vi "Signal generator (subVI).vi"(6 "DSA settings":T1={"function"=enum."Frequency response", "baseband span"=20000.0, "window"=enum."Hanning", "resolution (# of lines)"=800}, 7 "reset signal":bool, 8 "error in (no error)":errorcluster, 11 "signal generator":T2={"signal type"=enum."Uniform White noise", "frequency"=200.0, "amplitude"=1.0}) -> (0 "error out":errorcluster, 3 "signal out":waveform(dbl))   [LabVIEW 2020]
doc: "Generate typical test signal from the following choices: Sine wave, Square wave, Triangle wave, Sawtooth wave, Uniform White Noise, Gaussian White Noise, Periodic Random Noise (PRN), and Chirp."
uses:
  <vilib>/measure/NI_MABase.lvlib
  <vilib>/Analysis/NI_AALBase.lvlib
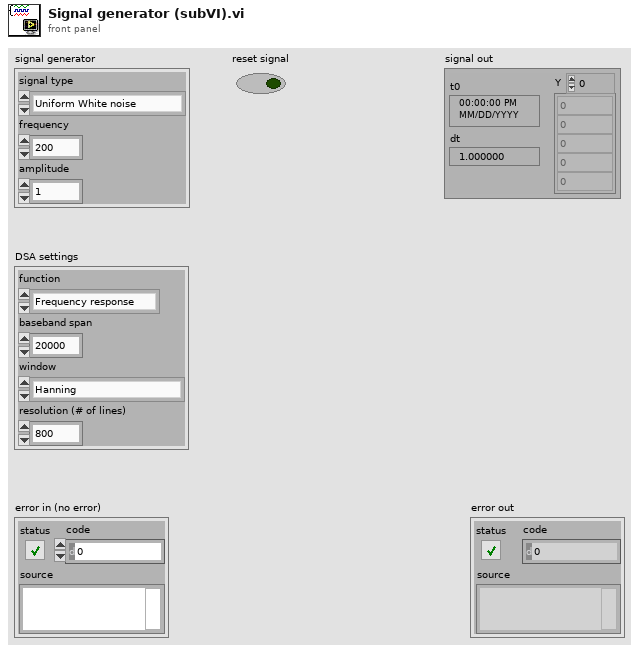
[diagram p1: front panel]
types:
  T1 = cluster{"function":enum16{"Windowed time", "Power Spectrum", "FFT (Mag-Phase)", "Cross Power spectrum", "Frequency response"}, "baseband span":dbl, "window":enum16{"None ", "Hanning", "Hamming", "Blackman-Harris", "Exact Blackman", "Blackman", "Flat Top", "4 Term B-Harris ", "7 Term B-Harris", "Low Sidelobe"}, "resolution (# of lines)":u32}
  T2 = cluster{"signal type":enum16{"Sine", "Square", "Triangle", "Sawtooth", "Chirp", "Uniform White noise", "Gaussian white noise", "PRN"}, "frequency":dbl, "amplitude":dbl}
  T3 = enum16{"Sine", "Square", "Triangle", "Sawtooth", "Chirp", "Uniform White noise", "Gaussian white noise", "PRN"}
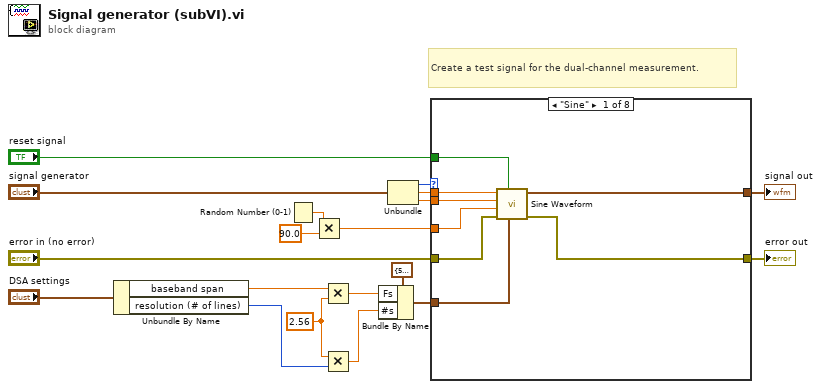
[diagram p0: block diagram]
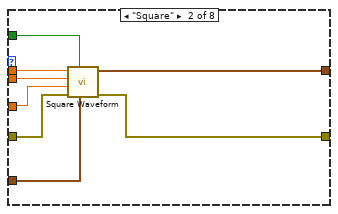
[diagram p2: hidden frame]
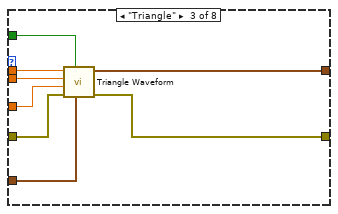
[diagram p3: hidden frame]
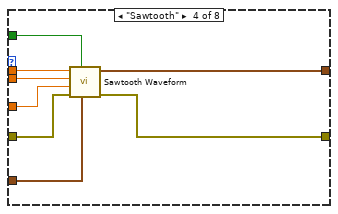
[diagram p4: hidden frame]
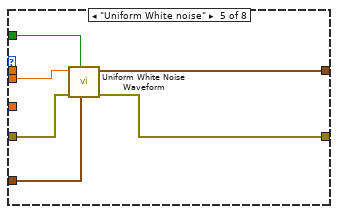
[diagram p5: hidden frame]
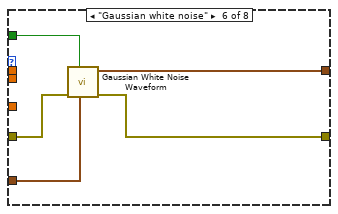
[diagram p6: hidden frame]
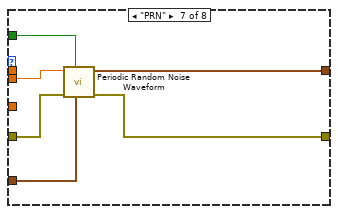
[diagram p7: hidden frame]
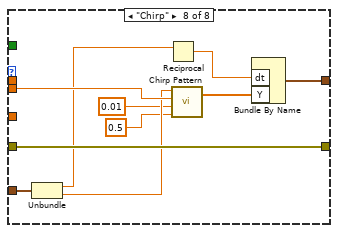
[diagram p8: hidden frame]
diagram:
  w3 = 2.56 ("y")
  # "Create a test signal for the dual-channel measurement."
  n1 = Unbundle By Name("DSA settings") -> ("baseband span"=w11:dbl, "resolution (# of lines)"=w1:u32)
  n2 = Random Number (0-1)() -> (number: 0 to 1=w7:dbl)
  n3 = Multiply(x=w7, y=90.0) -> (x*y=w5:dbl)
  n4 = Multiply(x=w11, y=w3) -> (x*y=w8:dbl)
  n5 = Multiply(x=w3, y=w1) -> (x*y=w2:dbl)
  n6 = Bundle By Name(cluster=cluster{"Fs":dbl, "#s":dbl} {"Fs"=51200.0, "#s"=1024.0} ("sampling info"), "Fs"=w8, "#s"=w2) -> (w10:cluster{"Fs":dbl, "#s":dbl})
  n7 = Unbundle("signal generator") -> ("signal type"=w9:T3, "frequency"=w15:dbl, "amplitude"=w14:dbl)
  n8 = case shown="\"Sine\"" w9 {
    tunnel: [w27 w35 w43 w51 w57 w62 w68 w75] -> w17
    tunnel: [w26 w34 w42 w50 w56 w61 w67 w78] -> w19
    tunnel: w15 -> [w25 w33 w41 w49 _ _ _ _]
    tunnel: w14 -> [w24 w31 w40 w48 w55 _ w65 w77]
    tunnel: "error in (no error)" -> [w23 w32 w39 w47 w54 w60 w66 w78]
    tunnel: w10 -> [w22 w30 w38 w46 w53 w59 w64 w73]
    tunnel: w5 -> [w21 w29 w37 w45 _ _ _ _]
    tunnel: "reset signal" -> [w20 w28 w36 w44 w52 w58 w63 _]
    frame "Sine" {
      n9 = call <vilib>:"Sine Waveform.vi"("sampling info"=w22, "reset signal"=w20, "error in (no error)"=w23, "phase"=w21, "amplitude"=w24, "frequency"=w25) -> ("error out"=w26:errorcluster, "signal out"=w27:waveform(dbl))  [unwired: 4 in]
    }
    frame "Square" {
      n10 = call <vilib>:"Square Waveform.vi"("sampling info"=w30, "reset signal"=w28, "error in (no error)"=w32, "phase"=w29, "amplitude"=w31, "frequency"=w33) -> ("error out"=w34:errorcluster, "signal out"=w35:waveform(dbl))  [unwired: 4 in]
    }
    frame "Triangle" {
      n11 = call <vilib>:"Triangle Waveform.vi"("sampling info"=w38, "reset signal"=w36, "error in (no error)"=w39, "phase"=w37, "amplitude"=w40, "frequency"=w41) -> ("error out"=w42:errorcluster, "signal out"=w43:waveform(dbl))  [unwired: 4 in]
    }
    frame "Sawtooth" {
      n12 = call <vilib>:"Sawtooth Waveform.vi"("sampling info"=w46, "reset signal"=w44, "error in (no error)"=w47, "phase"=w45, "amplitude"=w48, "frequency"=w49) -> ("error out"=w50:errorcluster, "signal out"=w51:waveform(dbl))  [unwired: 4 in]
    }
    frame "Uniform White noise" {
      n13 = call <vilib>:"Uniform White Noise Waveform.vi"("sampling info"=w53, "reset signal"=w52, "error in (no error)"=w54, "amplitude"=w55) -> ("error out"=w56:errorcluster, "signal out"=w57:waveform(dbl))  [unwired: 6 in]
    }
    frame "Gaussian white noise" {
      n14 = call <vilib>:"Gaussian White Noise Waveform.vi"("sampling info"=w59, "reset signal"=w58, "error in (no error)"=w60) -> ("error out"=w61:errorcluster, "signal out"=w62:waveform(dbl))  [unwired: 7 in]
    }
    frame "PRN" {
      n15 = call <vilib>:"Periodic Random Noise Waveform.vi"("sampling info"=w64, "reset signal"=w63, "error in (no error)"=w66, "spectral amplitude"=w65) -> ("error out"=w67:errorcluster, "signal out"=w68:waveform(dbl))  [unwired: 6 in]
    }
    frame "Chirp" {
      n16 = Unbundle(w73) -> ("Fs"=w72:dbl, "#s"=w71:dbl)
      n17 = Reciprocal(x=w72) -> (1/x=w74:dbl)
      n18 = call <vilib>:"Chirp Pattern.vi"("f2"=0.5, "f1"=0.01, "amplitude"=w77, "samples"=w71) -> ("Chirp Pattern"=w76:dbl[])  [unwired: 1 out]
      n19 = Bundle By Name("dt"=w74, "Y"=w76) -> (w75:waveform(dbl))  [unwired: 1 in]
    }
  }
  "error out" <- w19
  "signal out" <- w17
